vi "configure.vi"(8 "error in (no error)":errorcluster, 9 "Serial Message Parameters":T1={"Byte Count"=200, "Enable Termination Character"=FALSE, "Termination Char"=200} {"Termination Char" format="%x"}, 10 "Protocol Parameters":T2={"VISA resource name"="", "Baud Rate"=9600, "Data Bits"=8, "Parity"=enum."None", "Flow Control"=0, "Stop Bits"=10, "Timeout (ms)"=10000} {"Stop Bits" items=["1.0"=10, "1.5"=15, "2.0"=20]; "Flow Control" items=["None", "XON/XOFF", "RTS/CTS", "XON/XOFF & RTS/CTS", "DTR/DSR", "XON/XOFF & DTR/DSR"]; "Data Bits" min=5 max=8 step=1}, 11 "SerialSimulator in":refnum<class "SerialSimulator.lvclass">) -> (0 "error out":errorcluster, 3 "SerialSimulator out":refnum<class "SerialSimulator.lvclass">)   [LabVIEW 2013, in "SerialProtocols.lvlib" / "SerialSimulator.lvclass"]
uses:
  <userlib>/Common/SerialProtocols/SerialProtocol/SerialSimulator/SerialSimulator.lvclass
  <userlib>/Common/SerialProtocols/Configuration/ProtocolParameters.ctl
  <userlib>/Common/SerialProtocols/Configuration/SerialMessageParameters.ctl
  <userlib>/Common/SerialProtocols/SerialProtocol/SerialSimulator/SerialSimulator.lvclass/SerialSimulator.ctl
  LSST_TS/SystemSW/M2AADT/SimulateSerialData/SimulateSerialData/SimulateSerialData.lvclass
  <userlib>/Common/SerialProtocols/SerialProtocols.lvlib
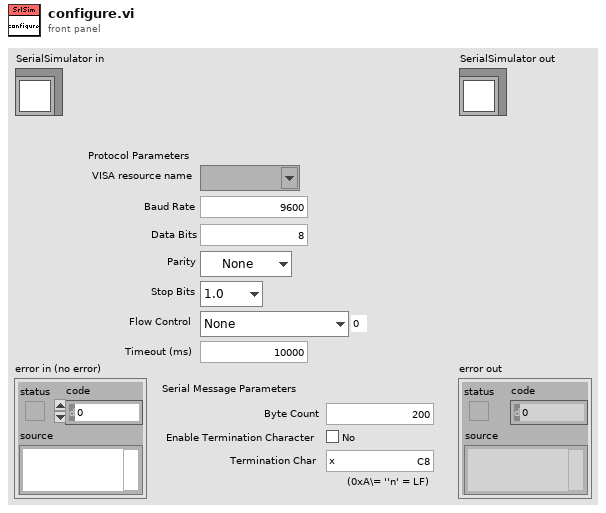
[diagram p1: front panel]
types:
  T1 = typedef "SerialProtocols.lvlib/SerialMessageParameters.ctl" = cluster{"Byte Count":u32, "Enable Termination Character":bool, "Termination Char":u8}
  T2 = typedef "SerialProtocols.lvlib/ProtocolParameters.ctl" = cluster{"VISA resource name":refnum<visa-resource-name>, "Baud Rate":u32, "Data Bits":u16, "Parity":enum16{"None", "Odd", "Even", "Mark", "Space"}, "Flow Control":u16, "Stop Bits":u16, "Timeout (ms)":u32}
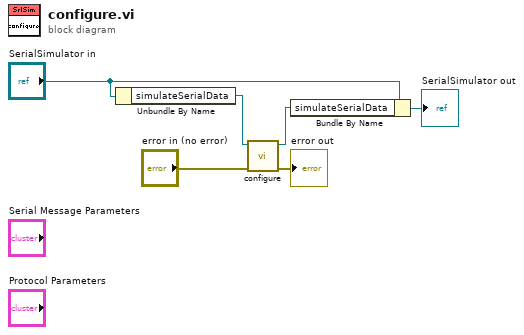
[diagram p0: block diagram]
diagram:
  n1 = Unbundle By Name("SerialSimulator in") -> ("simulateSerialData"=w5:refnum<class "SimulateSerialData.lvclass">)
  n2 = call-dynamic "configure.vi"("error in (no error)"="error in (no error)", "SimulateSerialData in"=w5) -> ("error out"=→"error out":errorcluster, "SimulateSerialData out"=w4:refnum<class "SimulateSerialData.lvclass">)  [unwired: 8 in]
  n3 = Bundle By Name(cluster="SerialSimulator in", "simulateSerialData"=w4) -> (→"SerialSimulator out":refnum<class "SerialSimulator.lvclass">)
